vi "Check Node Class Name.vi"(8 "error in (no error)":errorcluster, 10 "Node Path":string, 11 "FPGADMAChannelData in":refnum<class "FPGADMAChannelData.lvclass">) -> (0 "error out":errorcluster, 1 "Found Class?":bool, 2 "Node*":refnum<data-value>, 3 "FPGADMAChannelData out":refnum<class "FPGADMAChannelData.lvclass">)   [LabVIEW 2013, in "FPGADMAChannelData.lvclass"]
uses:
  FPGADMAChannelData.lvclass
  xCE/xceNode/xceNode.lvclass
  xCE/xceDataNode/xceDataNode.lvclass
  XML Parser/XML Parser.lvclass
panel:
  in  "Node Class Filter":string[](array[string])=["DMA_Read", "DMA_Write", "Packet"]
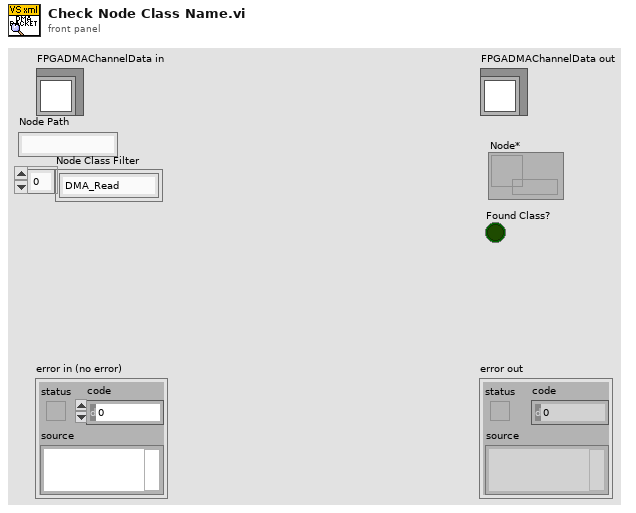
[diagram p1: front panel]
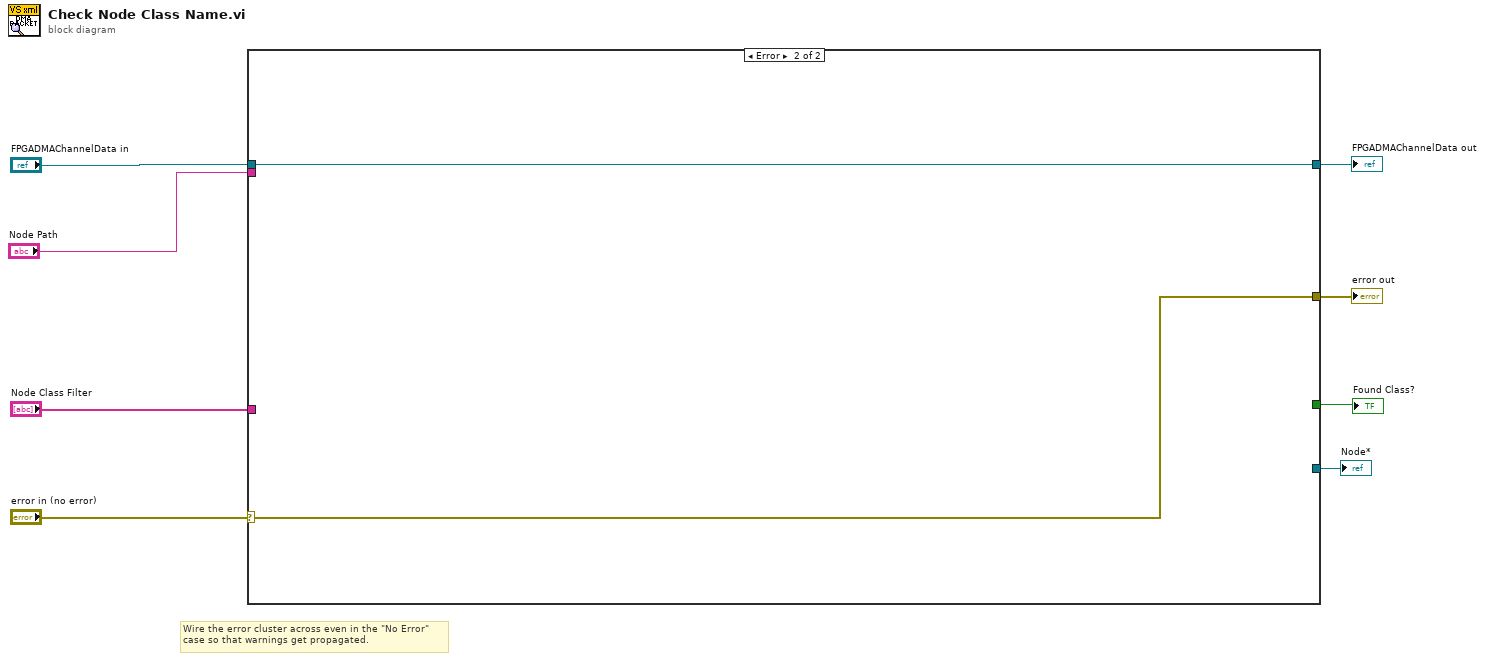
[diagram p0: block diagram]
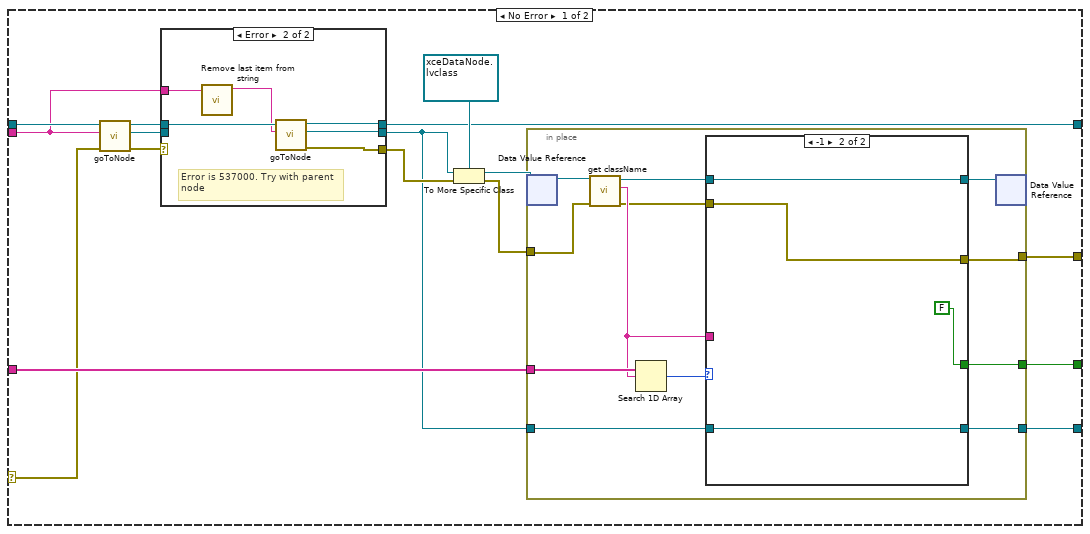
[diagram p2: hidden frame]
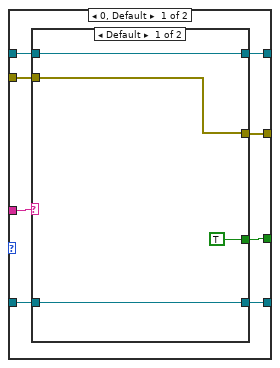
[diagram p4: hidden frame]
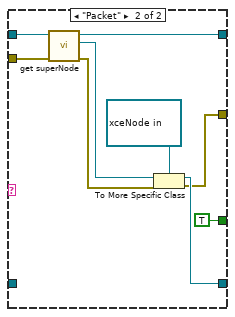
[diagram p5: hidden frame]
diagram:
  # "Wire the error cluster across even in the \"No Error\"\ncase so that warnings get propagated."
  n1 = case shown="Error" "error in (no error)" {
    selector: "error in (no error)" -> [w20 w72]
    tunnel: [w12 w72] -> w7
    tunnel: [w17 w71] -> w5
    tunnel: "FPGADMAChannelData in" -> [w21 w71]
    tunnel: "Node Class Filter" -> [w22 _]
    tunnel: "Node Path" -> [w13 _]
    tunnel: [w10 _] -> w2
    tunnel: [w9 _] -> w1
    frame No Error {
      n2 = call "goToNode.vi"("error in (no error)"=w20, "Node Path"=w13, "xceNode in"=w21) -> ("error out"=w18:errorcluster, "goToNode* out"=w14:refnum<data-value>, "xceNode out"=w16:refnum<class "FPGADMAChannelData.lvclass">)  [unwired: 6 in]
      n3 = case shown="Error" w18 {
        selector: w18 -> [w26 _]
        tunnel: [w27 w33] -> w17
        tunnel: w16 -> [w27 w32]
        tunnel: [w26 w30] -> w15
        tunnel: [w25 w31] -> w11
        tunnel: w14 -> [w25 _]
        tunnel: w13 -> [_ w29]
        frame No Error {
        }
        frame Error {
          # "Error is 537000. Try with parent\nnode"
          n4 = call "Remove last item from string.vi"("String"=w29) -> ("String w/o item"=w28:string)  [unwired: 9 in, 1 out]
          n5 = call "goToNode.vi"("Node Path"=w28, "xceNode in"=w32) -> ("error out"=w30:errorcluster, "goToNode* out"=w31:refnum<data-value>, "xceNode out"=w33:refnum<class "FPGADMAChannelData.lvclass">)  [unwired: 7 in]
        }
      }
      n6 = To More Specific Class(target class=refnum<data-value> refnum ("data value reference"), reference=w11, error in=w15) -> (specific class reference=w24:refnum<data-value>, error out=w23:errorcluster)
      n7 = in-place {
        in-place-border: w23 -> [w44]
        in-place-border: w22 -> [w43]
        in-place-border: [w35] -> w12
        in-place-border: w11 -> [w42]
        in-place-border: [w39] -> w10
        in-place-border: [w38] -> w9
        n8 = in-place-dvr #1(w24) -> (w45:refnum<class "xceDataNode.lvclass">)  [unwired: 1 out]
        n9 = call "get className.vi"("error in (no error)"=w44, "xceNode in"=w45) -> ("error out"=w36:errorcluster, "Class name"=w40:string, "xceNode out"=w37:refnum<class "xceDataNode.lvclass">)  [unwired: 7 in]
        n10 = Search 1D Array(1D array=w43, element=w40) -> (index of element=w41:i32)  [unwired: 1 in]
        n11 = case shown="-1" w41 {
          tunnel: w42 -> [w51 w70]
          tunnel: w40 -> [w53 _]
          tunnel: [w52 w70] -> w39
          tunnel: [w50 FALSE ("Found Class?")] -> w38
          tunnel: w37 -> [w49 w68]
          tunnel: w36 -> [w48 w67]
          tunnel: [w46 w67] -> w35
          tunnel: [w47 w68] -> w34
          frame 0, Default {
            n12 = case shown="Default" w53 {
              tunnel: [w57 w60] -> w52
              tunnel: w51 -> [w57 _]
              tunnel: [TRUE ("Found Class?") TRUE ("Found Class?")] -> w50
              tunnel: w49 -> [w55 w65]
              tunnel: w48 -> [w54 w64]
              tunnel: [w55 w59] -> w47
              tunnel: [w54 w58] -> w46
              frame Default {
              }
              frame "Packet" {
                n13 = call "get superNode.vi"("error in (no error)"=w64, "xceNode in"=w65) -> ("error out"=w62:errorcluster, "superNode*"=w61:refnum<data-value>, "xceNode out"=w59:refnum<class "xceDataNode.lvclass">)  [unwired: 7 in]
                n14 = To More Specific Class(target class=refnum<data-value> refnum ("goToNode* out"), reference=w61, error in=w62) -> (specific class reference=w60:refnum<data-value>, error out=w58:errorcluster)
              }
            }
          }
          frame -1 {
          }
        }
        n15 = in-place-dvr #1(w34) -> ()  [unwired: 2 out]
      }
    }
    frame Error {
    }
  }
  "error out" <- w7
  "FPGADMAChannelData out" <- w5
  "Node*" <- w2
  "Found Class?" <- w1
